vi "Random Graph Generator - Populate Boolean Transition Array.vi"(6 "1 to 0":bool=TRUE, 10 "Offset":dbl, 11 "Array Size":dbl) -> (3 "Array":dbl[](array[numeric]))   [LabVIEW 2021]
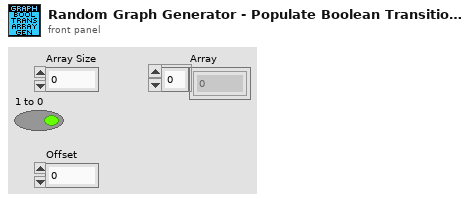
[diagram p1: front panel]
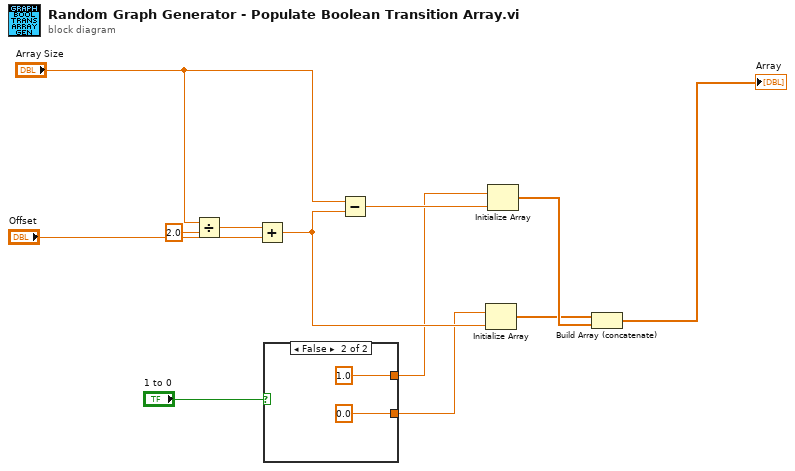
[diagram p0: block diagram]
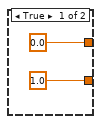
[diagram p2: hidden frame]
diagram:
  n1 = Divide(x="Array Size", y=2.0) -> (x/y=w10:dbl)
  n2 = Add(x=w10, y="Offset") -> (x+y=w11:dbl)
  n3 = case shown="False" "1 to 0" {
    tunnel: [0.0 ("element") 1.0 ("element")] -> w4
    tunnel: [1.0 ("element") 0.0 ("element")] -> w3
    frame True {
    }
    frame False {
    }
  }
  n4 = Subtract(x="Array Size", y=w11) -> (x-y=w6:dbl)
  n5 = Initialize Array(w3, w11) -> (w7:dbl[])
  n6 = Initialize Array(w4, w6) -> (w8:dbl[])
  n7 = Build Array (concatenate)(w7, w8) -> (→"Array":dbl[])
